vi "Coerce Cutoff Frequency Controls.vi"(8 "Sampling Frequency":dbl, 9 "Filter Type":refnum<vi>, 10 "High Cutoff Frequency":refnum<vi>, 11 "Low Cutoff Frequency":refnum<vi>) -> ()   [LabVIEW 2014]
uses:
  <vilib>/Utility/miscctls.llb/LVOutOfRangeActionTypeDef.ctl
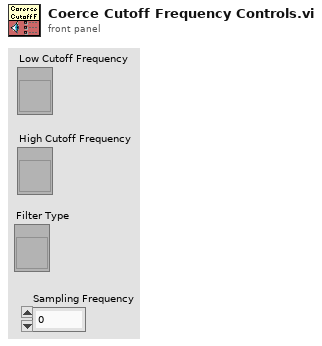
[diagram p1: front panel]
types:
  T1 = typedef "LVOutOfRangeActionTypeDef.ctl" = cluster{"Out of Range Action Minimum":u8, "Out of Range Action Maximum":u8, "Out of Range Action Increment":u8}
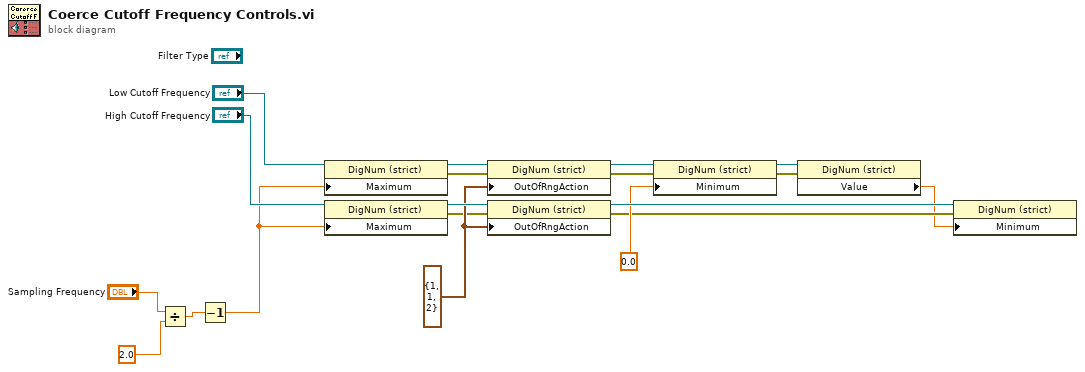
[diagram p0: block diagram]
diagram:
  w9 = T1 {"Out of Range Action Minimum"=1, "Out of Range Action Maximum"=1, "Out of Range Action Increment"=2} ("Response to Value Outside Limits")
  n1 = Divide(x="Sampling Frequency", y=2.0) -> (x/y=w13:dbl)
  n2 = Decrement(x=w13) -> (x-1=w15:dbl)
  n3 = property class="DigNum (strict)"(reference="Low Cutoff Frequency", "Maximum"=w15) -> (reference out=w17:refnum<vi>, error out=w5:errorcluster)  [unwired: 1 in]
  n4 = property class="DigNum (strict)"(reference="High Cutoff Frequency", "Maximum"=w15) -> (reference out=w16:refnum<vi>, error out=w4:errorcluster)  [unwired: 1 in]
  n5 = property class="DigNum (strict)"(reference=w17, error in=w5, "OutOfRngAction"=w9) -> (reference out=w11:refnum<vi>, error out=w2:errorcluster)
  n6 = property class="DigNum (strict)"(reference=w16, error in=w4, "OutOfRngAction"=w9) -> (reference out=w10:refnum<vi>, error out=w3:errorcluster)
  n7 = property class="DigNum (strict)"(reference=w11, error in=w2, "Minimum"=0.0 ("Data Entry Limits:Minimum")) -> (reference out=w7:refnum<vi>, error out=w6:errorcluster)
  n8 = property class="DigNum (strict)"(reference=w7, error in=w6) -> ("Value"=w1:dbl)  [unwired: 2 out]
  n9 = property class="DigNum (strict)"(reference=w10, error in=w3, "Minimum"=w1) -> ()  [unwired: 2 out]
